vi "Init (Name).vi"(6 "Name":string, 8 "error in (no error)":errorcluster) -> (0 "error out":errorcluster, 2 "New":bool=TRUE, 3 "Carya Config (Buffer) out":refnum<class "CConfig By Ref Buffer.lvclass">)   [LabVIEW 2013, in "CConfig By Ref Buffer.lvclass"]
doc: "Copyright 2018, Carya Automatisering, Wiebe Walstra."
uses:
  CConfig By Ref Buffer.lvclass
  Buffer Functions.ctl
  CConfig By Ref Buffer.lvclass/CConfig By Ref Buffer.ctl
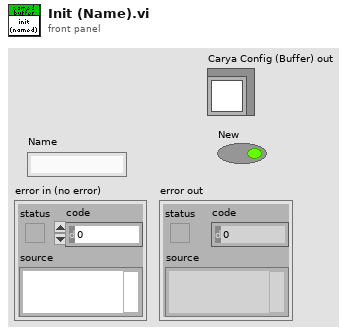
[diagram p1: front panel]
types:
  T1 = typedef "CConfig By Ref Buffer.lvclass/Buffer Functions.ctl" = enum16{"register", "get and lock", "set and unlock", "unlock", "unregister", "check"}
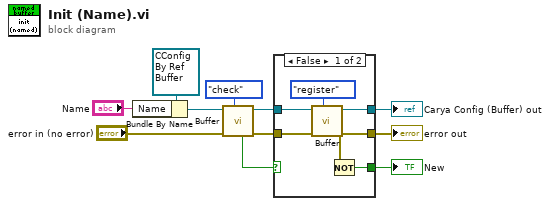
[diagram p0: block diagram]
diagram:
  n1 = Bundle By Name(cluster=refnum<class "CConfig By Ref Buffer.lvclass"> refnum ("Carya Config (Buffer) in"), "Name"="Name") -> (w7:refnum<class "CConfig By Ref Buffer.lvclass">)
  n2 = call "Buffer.vi"("Functions"=Buffer_Functions."check", "error in (no error)"="error in (no error)", "Carya Config (Buffer) in"=w7) -> ("error out"=w4:errorcluster, "Carya Config (Buffer) out"=w6:refnum<class "CConfig By Ref Buffer.lvclass">, "Wait\\Check"=w3:bool)  [unwired: 4 in, 2 out]
  n3 = case shown="False" w3 {
    tunnel: [w17 w19] -> w11
    tunnel: w6 -> [w15 w19]
    tunnel: w4 -> [w14 w18]
    tunnel: [w13 w18] -> w2
    tunnel: [w12 _] -> w1
    frame False {
      n4 = call "Buffer.vi"("Functions"=Buffer_Functions."register", "error in (no error)"=w14, "Carya Config (Buffer) in"=w15) -> ("error out"=w13:errorcluster, "Carya Config (Buffer) out"=w17:refnum<class "CConfig By Ref Buffer.lvclass">)  [unwired: 4 in, 3 out]
      n5 = Not(x=w13) -> (.not. x?=w12:bool)
    }
    frame True {
    }
  }
  "error out" <- w2
  "Carya Config (Buffer) out" <- w11
  "New" <- w1
